vi "Write TCP Connection.vi"(8 "error in (no error)":errorcluster, 10 "TCP Connection":refnum<k5>, 11 "MB_TCP_Device in":refnum<class "MB_TCP_Device.lvclass">) -> (0 "error out":errorcluster, 3 "MB_TCP_Device out":refnum<class "MB_TCP_Device.lvclass">)   [LabVIEW 2023, in "MB_TCP_Device.lvclass"]
uses:
  MB_TCP_Device.lvclass
  MB_TCP_Device.lvclass/MB_TCP_Device.ctl
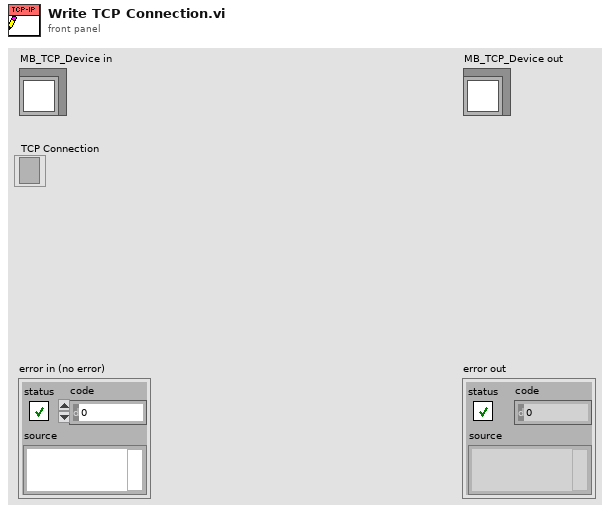
[diagram p1: front panel]
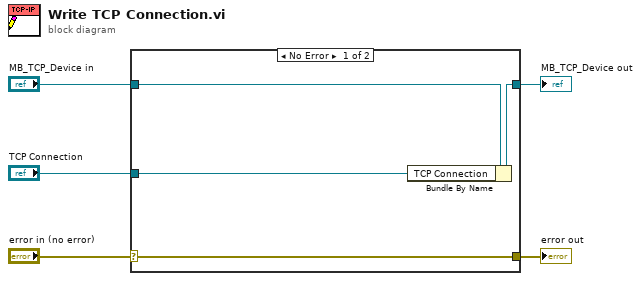
[diagram p0: block diagram]
diagram:
  n1 = case shown="No Error" "error in (no error)" {
    selector: "error in (no error)" -> [w9 w10]
    tunnel: [w9 w10] -> w4
    tunnel: [w7 w11] -> w2
    tunnel: "MB_TCP_Device in" -> [w8 w11]
    tunnel: "TCP Connection" -> [w6 _]
    frame No Error {
      n2 = Bundle By Name(cluster=w8, "TCP Connection"=w6) -> (w7:refnum<class "MB_TCP_Device.lvclass">)
    }
    frame Error {
    }
  }
  "error out" <- w4
  "MB_TCP_Device out" <- w2
